vi "MetaClientCont.vi"(8 "error in (no error)":errorcluster, 11 "Action":enum16{"Run", "Exit"}(ring)) -> (0 "error out":errorcluster, 3 "ContServerDataOut":string)   [LabVIEW 2019]
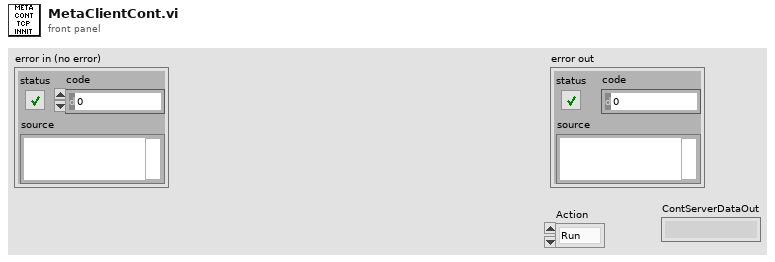
[diagram p1: front panel]
types:
  T1 = enum16{"Standard", "Buffered", "CRLF", "Immediate"}
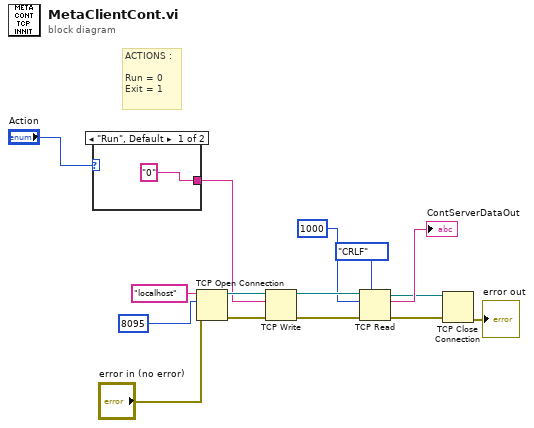
[diagram p0: block diagram]
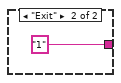
[diagram p2: hidden frame]
diagram:
  # "ACTIONS :\n\nRun = 0\nExit = 1"
  n1 = case shown="\"Run\", Default" "Action" {
    tunnel: ["0" "1"] -> w8
    frame "Run", Default {
    }
    frame "Exit" {
    }
  }
  n2 = TCP Open Connection(address="localhost", remote port or service name=u16 8095, error in (no error)="error in (no error)") -> (connection ID=w12:refnum<k5>, error out=w15:errorcluster)  [unwired: 2 in]
  n3 = TCP Write(connection ID=w12, data in=w8, error in (no error)=w15) -> (connection ID out=w13:refnum<k5>, error out=w14:errorcluster)  [unwired: 1 in, 1 out]
  n4 = TCP Read(connection ID=w13, bytes to read=1000, error in (no error)=w14, 7:T1."CRLF" ("mode (standard)")) -> (connection ID out=w3:refnum<k5>, data out=→"ContServerDataOut":string, error out=w4:errorcluster)  [unwired: 1 in]
  n5 = TCP Close Connection(connection ID=w3, error in (no error)=w4) -> (error out=→"error out":errorcluster)  [unwired: 1 in, 1 out]
